vi "User Interface.vi"(8 "error in (no error)":errorcluster, 11 "User Interface in":refnum<class "User Interface.lvclass">) -> (0 "error out":errorcluster, 3 "User Interface out":refnum<class "User Interface.lvclass">)   [LabVIEW 2019, in "DSF Core.lvlib" / "Core Thread User Interface.lvclass"]
uses:
  Core Thread User Interface.lvclass
  User Interface.lvclass
  Configuration/Core/Thread/Thread Configuration.lvclass
  C:/Dev/GitHub/niveristand-data-sharing-framework-custom-device/Core/Classes/Configuration/Configuration.lvclass
  Configuration/Configuration.lvclass
panel:
  in  "Priority Offset":i16
  in  "Processor":i32=-2
  out "Data Version":string
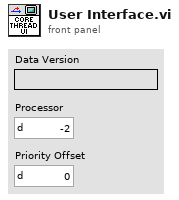
[diagram p1: front panel]
types:
  T1 = typedef "DSF Core.lvlib/Thread Configuration.lvclass/Core Thread Configuration.ctl" = cluster{"processor":i32, "priority offset":i16}
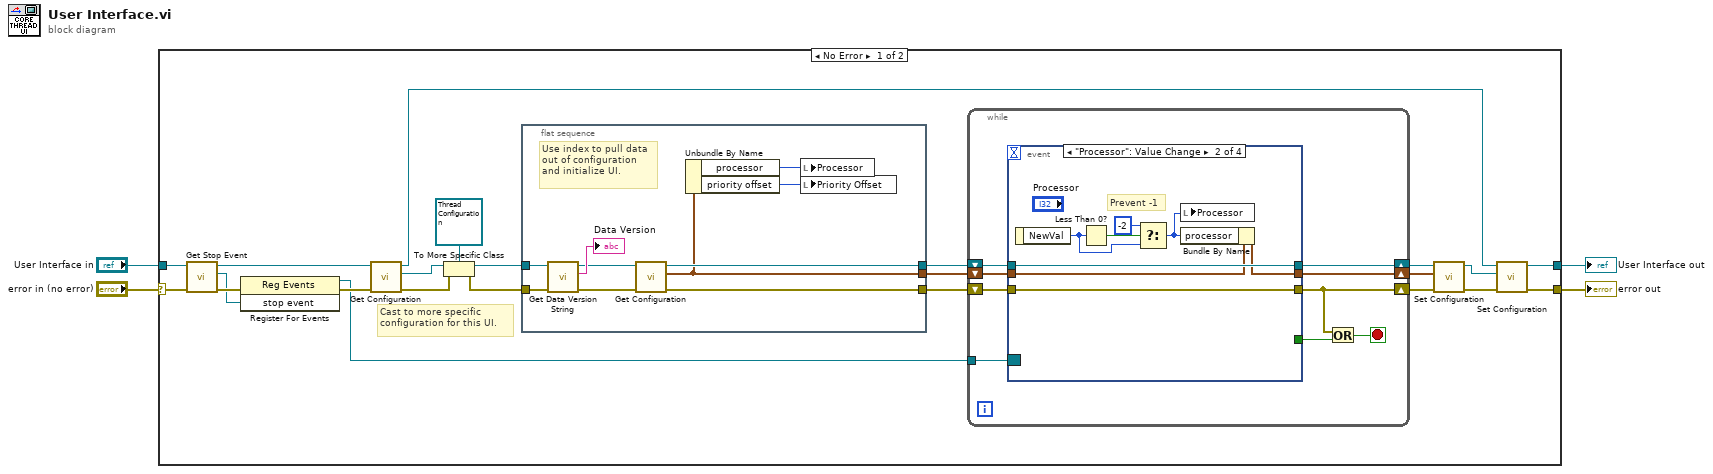
[diagram p0: block diagram]
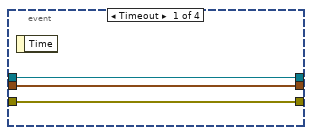
[diagram p2: hidden frame]
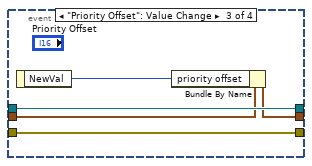
[diagram p3: hidden frame]
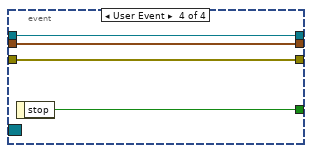
[diagram p4: hidden frame]
diagram:
  n1 = case shown="No Error" "error in (no error)" {
    selector: "error in (no error)" -> [w21 w68]
    tunnel: [w12 w68] -> w4
    tunnel: "User Interface in" -> [w22 w67]
    tunnel: [w11 w67] -> w1
    frame No Error {
      # "Cast to more specific configuration for this UI."
      n2 = call "Get Stop Event.vi"("error in (no error)"=w21, "User Interface in"=w22) -> ("error out"=w20:errorcluster, "stop event"=w19:refnum<user-event>, "User Interface out"=w18:refnum<class "User Interface.lvclass">)  [unwired: 7 in]
      n3 = register-events(error in=w20, w19) -> (reference out=w16:refnum<event-registration>, error out=w17:errorcluster)  [unwired: 1 in]
      n4 = call "Get Configuration.vi"("error in (no error)"=w17, "User Interface in"=w18) -> ("error out"=w15:errorcluster, "configuration"=w14:refnum<class "Configuration.lvclass">, "User Interface out"=w13:refnum<class "User Interface.lvclass">)  [unwired: 7 in]
      n5 = To More Specific Class(target class=refnum<class "Thread Configuration.lvclass"> refnum ("DSF Core.lvlib:Thread Configuration.lvclass"), reference=w14, error in=w15) -> (specific class reference=w27:refnum<class "Thread Configuration.lvclass">, error out=w24:errorcluster)
      n6 = flat-sequence {
        tunnel: [w30] -> w25
        tunnel: w24 -> [w37]
        tunnel: w27 -> [w36]
        tunnel: [w29] -> w26
        tunnel: [w28] -> w23
        frame #0 {
          # "Use index to pull data out of configuration and initialize UI."
          n7 = call "Get Data Version String.vi"("error in (no error)"=w37, "Configuration in"=w36) -> ("error out"=w31:errorcluster, "data version"=→"Data Version":string, "Configuration out"=w32:refnum<class "Thread Configuration.lvclass">)  [unwired: 7 in]
          n8 = call "Get Configuration.vi"("error in (no error)"=w31, "Core Threads Configuration in"=w32) -> ("error out"=w30:errorcluster, "configuration"=w28:T1, "Core Threads Configuration out"=w29:refnum<class "Thread Configuration.lvclass">)  [unwired: 7 in]
          n9 = Unbundle By Name(w28) -> ("processor"=w33:i32, "priority offset"=w34:i16)
          n10 = local write "Processor"(w33) -> ()
          n11 = local write "Priority Offset"(w34) -> ()
        }
      }
      n12 = while {
        tunnel: w16 -> [w46]
        shift-right: [w44] -> w8
        shift-left: w25 -> [w45]
        shift-right: [w41] -> w9
        shift-left: w26 -> [w40]
        shift-right: [w38] -> w6
        shift-left: w23 -> [w39]
        stop <- w43 stop-if-true
        n13 = event shown="[1] \"Processor\": Value Change" {
          selector: w46 -> [_ _ _ _]
          dyn-events: _ -> [_ _ _ _]
          timeout: _ -> [_ _ _ _]
          tunnel: [_ _ _ w64] -> w42
          tunnel: w45 -> [w49 w57 w62 w66]
          tunnel: [w49 w57 w62 w66] -> w44
          tunnel: w40 -> [w48 w56 w61 w65]
          tunnel: [w48 w56 w61 w65] -> w41
          tunnel: w39 -> [w47 w54 w59 w63]
          tunnel: [w47 w55 w60 w63] -> w38
          event Timeout {
            n14 = event-data() -> ()  [unwired: 1 in, 1 out]
          }
          event "Processor": Value Change {
            # "Prevent -1"
            n15 = event-data() -> ("NewVal"=w51:i32)  [unwired: 1 in]
            n16 = Less Than 0?(x=w51) -> (x < 0?=w53:bool)
            n17 = Select(t=-2, s=w53, f=w51) -> (s? t:f=w50:i32)
            n18 = local write "Processor"(w50) -> ()
            n19 = Bundle By Name(cluster=w54, "processor"=w50) -> (w55:T1)
          }
          event "Priority Offset": Value Change {
            n20 = event-data() -> ("NewVal"=w58:i16)  [unwired: 1 in]
            n21 = Bundle By Name(cluster=w59, "priority offset"=w58) -> (w60:T1)
          }
          event User Event {
            n22 = event-data() -> ("stop"=w64:bool)  [unwired: 1 in]
          }
        }
        n23 = Or(x=w44, y=w42) -> (x .or. y?=w43:bool)
      }
      n24 = call "Set Configuration.vi"("error in (no error)"=w8, "configuration"=w6, "Core Threads Configuration in"=w9) -> ("error out"=w7:errorcluster, "Core Threads Configuration out"=w5:refnum<class "Thread Configuration.lvclass">)  [unwired: 7 in]
      n25 = call "Set Configuration.vi"("error in (no error)"=w7, "configuration"=w5, "User Interface in"=w13) -> ("error out"=w12:errorcluster, "User Interface out"=w11:refnum<class "User Interface.lvclass">)  [unwired: 7 in]
    }
    frame Error {
    }
  }
  "error out" <- w4
  "User Interface out" <- w1
